vi "Day 15.vi"() -> ()   [LabVIEW 2023]
panel:
  out "sum":i32
  in  "test":bool
  in  "test input":string="Sensor at x=2, y=18: closest beacon is at x=-2, y=15\nSensor at x=9, y=16: closest beacon is at x=10, y=16\nSensor at x=13, y=2: closest beacon is at x=15, y=3\nSensor at x=12, y=14: closest beacon is at x=10, y=16\nSensor at x=10, y=20: closest beacon is at x=10, y=16\nSensor at x=14, y=17: closest beacon is at x=10, y=16\nSensor at x=8, y=7: closest beacon is at x=2, y=10\nSensor at x=2, y=0: closest beacon is at x=2, y=10\nSensor at x=0, y=11: closest beacon is at x=2, y=10\nSensor at x=20, y=14: closest beacon is at x=25, y=17\nSensor at x=17, y=20: closest beacon is at x=21, y=22\nSensor at x=16, y=7: closest beacon is at x=15, y=3\nSensor at x=14, y=3: closest beacon is at x=15, y=3\nSensor at x=20, y=1: closest beacon is at x=15, y=3"
  in  "input":string="Sensor at x=3289936, y=2240812: closest beacon is at x=3232809, y=2000000\nSensor at x=30408, y=622853: closest beacon is at x=-669401, y=844810\nSensor at x=3983196, y=3966332: closest beacon is at x=3232807, y=4625568\nSensor at x=929672, y=476353: closest beacon is at x=-669401, y=844810\nSensor at x=1485689, y=3597734: closest beacon is at x=1951675, y=3073734\nSensor at x=69493, y=1886070: closest beacon is at x=-669401, y=844810\nSensor at x=2146060, y=3999371: closest beacon is at x=2300657, y=4128792\nSensor at x=3228558, y=3890086: closest beacon is at x=3232807, y=4625568\nSensor at x=3031444, y=2295853: closest beacon is at x=2928827, y=2611422\nSensor at x=374444, y=3977240: closest beacon is at x=-888612, y=4039783\nSensor at x=1207660, y=2710720: closest beacon is at x=1951675, y=3073734\nSensor at x=3851310, y=61626: closest beacon is at x=4807592, y=976495\nSensor at x=3195193, y=3022787: closest beacon is at x=2928827, y=2611422\nSensor at x=1784895, y=2111901: closest beacon is at x=1951675, y=3073734\nSensor at x=2894075, y=2427030: closest beacon is at x=2928827, y=2611422\nSensor at x=3301867, y=803327: closest beacon is at x=3232809, y=2000000\nSensor at x=2506616, y=3673347: closest beacon is at x=2300657, y=4128792\nSensor at x=2628426, y=3054377: closest beacon is at x=1951675, y=3073734\nSensor at x=2521975, y=1407505: closest beacon is at x=3232809, y=2000000\nSensor at x=2825447, y=2045173: closest beacon is at x=3232809, y=2000000\nSensor at x=2261212, y=2535886: closest beacon is at x=2928827, y=2611422\nSensor at x=3956000, y=1616443: closest beacon is at x=3232809, y=2000000\nSensor at x=3870784, y=2872668: closest beacon is at x=2928827, y=2611422\n"
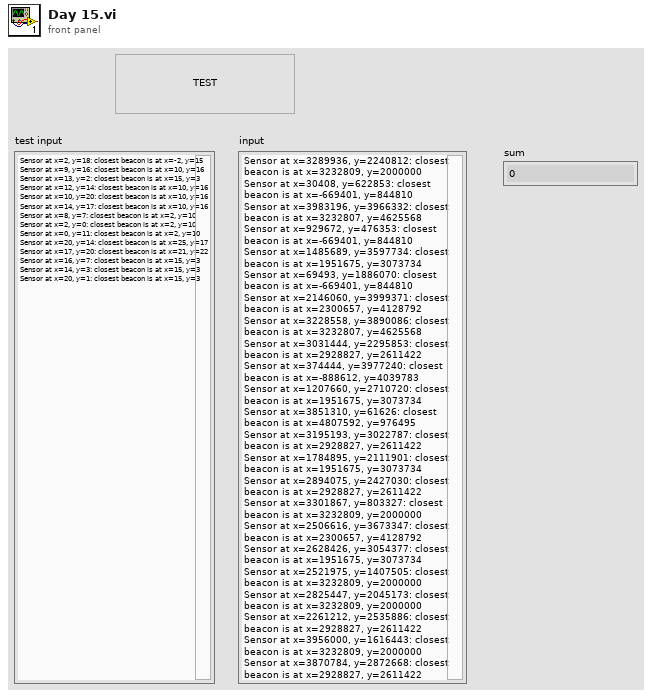
[diagram p1: front panel]
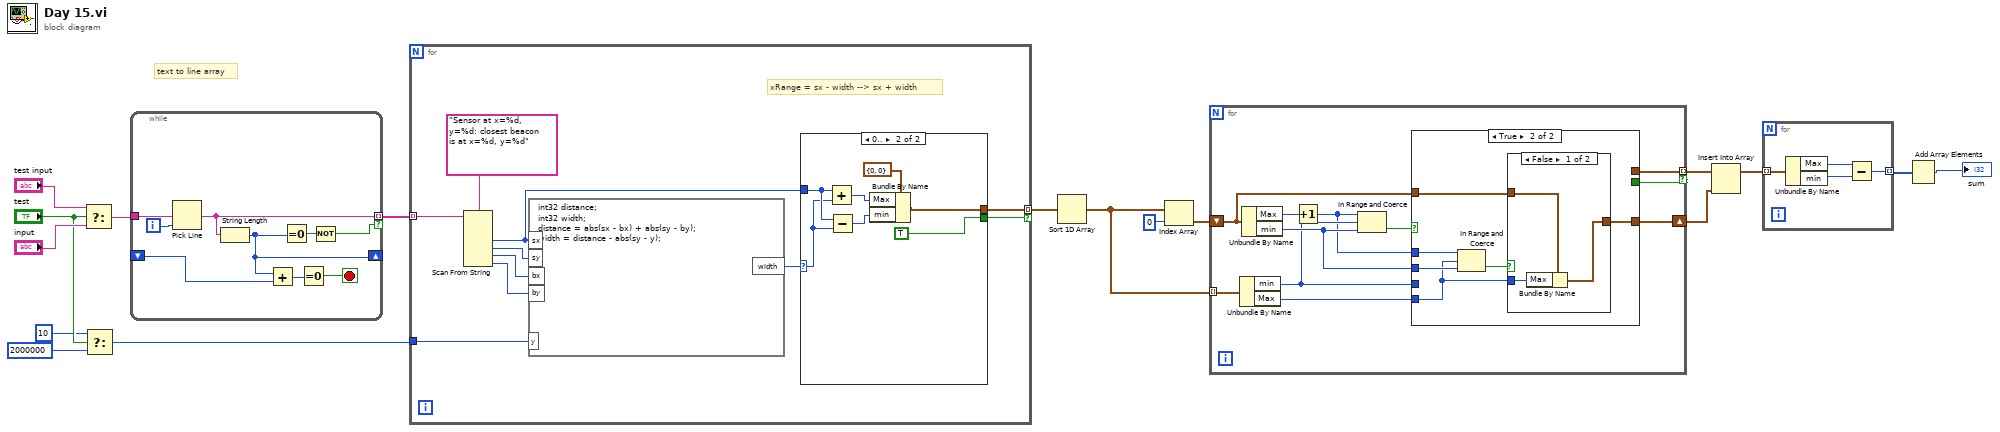
[diagram p0: block diagram]
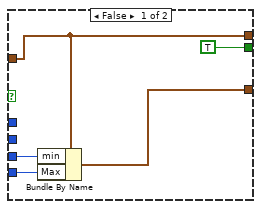
[diagram p3: hidden frame]
diagram:
  # "text to line array"
  n1 = Select(t="test input", s="test", f="input") -> (s? t:f=w14:string)
  n2 = Select(t=10 ("output 4"), s="test", f=2000000 ("output 4")) -> (s? t:f=w10:i32)
  n3 = while {
    tunnel: w14 -> [w25]
    tunnel: [w18] -> w15 mode=indexing if=w24
    shift-right: [w21] -> _
    shift-left: _ -> [w22]
    i -> [w26]
    stop <- w19 stop-if-true
    n4 = Pick Line(multi-line string=w25, line index=w26) -> (output string=w18:string)  [unwired: 1 in]
    n5 = String Length(string=w18) -> (length=w21:i32)
    n6 = Add(x=w21, y=w22) -> (x+y=w23:i32)
    n7 = Equal To 0?(x=w21) -> (x = 0?=w20:bool)
    n8 = Equal To 0?(x=w23) -> (x = 0?=w19:bool)
    n9 = Not(x=w20) -> (.not. x?=w24:bool)
  }
  n10 = for {
    tunnel: w15 -> [w36] mode=indexing
    tunnel: w10 -> [w31]
    tunnel: [w28] -> w9 mode=indexing if=w27
    # "xRange = sx - width --> sx + width"
    n11 = Scan From String(format string="Sensor at x=%d, y=%d: closest beacon is at x=%d, y=%d", input string=w36) -> (output 1=w29:i32, output 2=w34:i32, output 3=w33:i32, output 4=w32:i32)  [unwired: 6 in, 3 out]
    n12 = formula code="int32 distance;\nint32 width;\ndistance = abs(sx - bx) + abs(sy - by);\nwidth = distance - abs(sy - y);"("sx"=w29, "sy"=w34, "bx"=w33, "by"=w32, "y"=w31) -> ("width"=w30:i32)
    n13 = case shown="0.." w30 {
      selector: w30 -> [_ w42]
      tunnel: w29 -> [_ w43]
      tunnel: [_ w41] -> w28
      tunnel: [_ TRUE] -> w27
      frame -1, Default {
      }
      frame 0.. {
        n14 = Add(x=w43, y=w42) -> (x+y=w38:i32)
        n15 = Subtract(x=w43, y=w42) -> (x-y=w39:i32)
        n16 = Bundle By Name(cluster=cluster{"min":i32, "Max":i32} {"min"=0, "Max"=0} ("output cluster"), "Max"=w38, "min"=w39) -> (w41:cluster{"min":i32, "Max":i32})
      }
    }
  }
  n17 = Sort 1D Array(array=w9) -> (sorted array=w6:cluster{"min":i32, "Max":i32}[])
  n18 = Index Array(array=w6, index=0) -> (element=w5:cluster{"min":i32, "Max":i32})
  n19 = for {
    tunnel: w6 -> [w53] mode=indexing
    shift-right: [w48] -> w7
    shift-left: w5 -> [w49]
    tunnel: [w47] -> w8 mode=indexing if=w46
    n20 = Unbundle By Name(w53) -> ("min"=w45:i32, "Max"=w50:i32)
    n21 = Unbundle By Name(w49) -> ("Max"=w51:i32, "min"=w52:i32)
    n22 = Increment(x=w51) -> (x+1=w44:i32)
    n23 = In Range and Coerce(upper limit=w44, x=w45, lower limit=w52) -> (In Range?=w54:bool)  [unwired: 1 out]
    n24 = case shown="True" w54 {
      tunnel: w52 -> [_ w63]
      tunnel: w44 -> [_ w65]
      tunnel: w50 -> [w58 w61]
      tunnel: w49 -> [w55 w62]
      tunnel: [w56 w60] -> w48
      tunnel: [w55 _] -> w47
      tunnel: [TRUE _] -> w46
      tunnel: w45 -> [w57 _]
      frame False {
        n25 = Bundle By Name(cluster=w55, "min"=w57, "Max"=w58) -> (w56:cluster{"min":i32, "Max":i32})
      }
      frame True {
        n26 = In Range and Coerce(upper limit=w65, x=w61, lower limit=w63) -> (In Range?=w64:bool)  [unwired: 1 out]
        n27 = case shown="False" w64 {
          tunnel: w62 -> [w68 w69]
          tunnel: w61 -> [w67 _]
          tunnel: [w66 w69] -> w60
          frame False {
            n28 = Bundle By Name(cluster=w68, "Max"=w67) -> (w66:cluster{"min":i32, "Max":i32})
          }
          frame True {
          }
        }
      }
    }
  }
  n29 = Insert Into Array(array=w8, new element=w7) -> (w3:cluster{"min":i32, "Max":i32}[])  [unwired: 1 in]
  n30 = for {
    tunnel: w3 -> [w73] mode=indexing
    tunnel: [w70] -> w2 mode=indexing
    n31 = Unbundle By Name(w73) -> ("Max"=w72:i32, "min"=w71:i32)
    n32 = Subtract(x=w72, y=w71) -> (x-y=w70:i32)
  }
  n33 = Add Array Elements(numeric array=w2) -> (sum=→"sum":i32)
